vi "Dialog Condition Client.vi"() -> ()   [LabVIEW 2019, in "OPC UA Demo.lvlib"]
doc: "Demonstrates the use of the <B>OPC UA Dialog Condition</B> functionality as an OPC UA client."
uses:
  OPC UA Demo.lvlib
  <vilib>/OPCUA/controls/NodeIds.ctl
  <vilib>/OPCUA/controls/NodeId.ctl
  <vilib>/OPCUA/controls/Write Variant Request.ctl
  <vilib>/OPCUA/controls/Write Status.ctl
  <vilib>/OPCUA/client/Multiple Write Variant.vi
  <vilib>/OPCUA/NI OPC UA Client.lvlib
panel:
  in  "enable/disable":bool
  in  "source node ID":string="Notifier.Source Node"
  out "active":bool
  in  "condition node ID":string="ns=2;s=Notifier.Dialog Condition Node"
  in  "stop":bool
  in  "server endpoint URL":string="opc.tcp://localhost:49580"
  # "Overview: Demonstrates the use of the OPC UA Dialog Condition functionality as an OPC UA client.\nRequirements: \n1. LabVIEW OPC UA Toolkit\n2. Run this VI on RT targets or Windows\nInstructions:\n1. Specify the server endpoint URL generated by the server.\n2. Run the VI.\n3. Click enable/disable to enable/disable the dialog condition node."
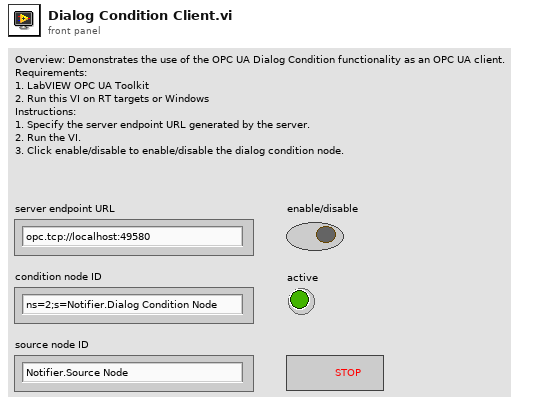
[diagram p1: front panel]
types:
  T1 = typedef "NodeIds.ctl" = T2[]
  T2 = typedef "NodeId.ctl" = string
  T3 = cluster{"message mode":enum16{"None", "Sign", "Sign and Encrypt"}, "security":enum16{"Basic256", "Basic128Rsa15"}}
  T4 = typedef "OPC UA Client Refnum.ctl" = refnum<k21>
  T5 = typedef "Subscription ID.ctl" = u32
  T6 = typedef "Write Variant Request.ctl" = cluster{"node ID":T2, "value":variant, "timestamp (current time)":timestamp, "node status":T7}
  T7 = typedef "Write Status.ctl" = u32
  T8 = typedef "Event Fields.ctl" = cluster{"condition node ID":T2, "condition type":T9, "source node ID/input node ID":T2, "event ID":string, "active":bool, "time":timestamp, "severity":u16, "quality":T10, "comment":string, "limit state":cluster{"high high state":bool, "high state":bool, "low state":bool, "low low state":bool}, "acked state":bool, "confirmed state":bool, "prompt":string}
  T9 = typedef "Condition Type.ctl" = enum16{"Dialog Condition", "Off-Normal Alarm", "Exclusive Level Alarm", "Exclusive Deviation Alarm", "Exclusive Rate of Change Alarm", "Nonexclusive Level Alarm", "Nonexclusive Deviation Alarm", "Nonexclusive Rate of Change Alarm", "Refresh Start Event", "Refresh End Event"}
  T10 = typedef "OPC UA StatusCode.ctl" = u32
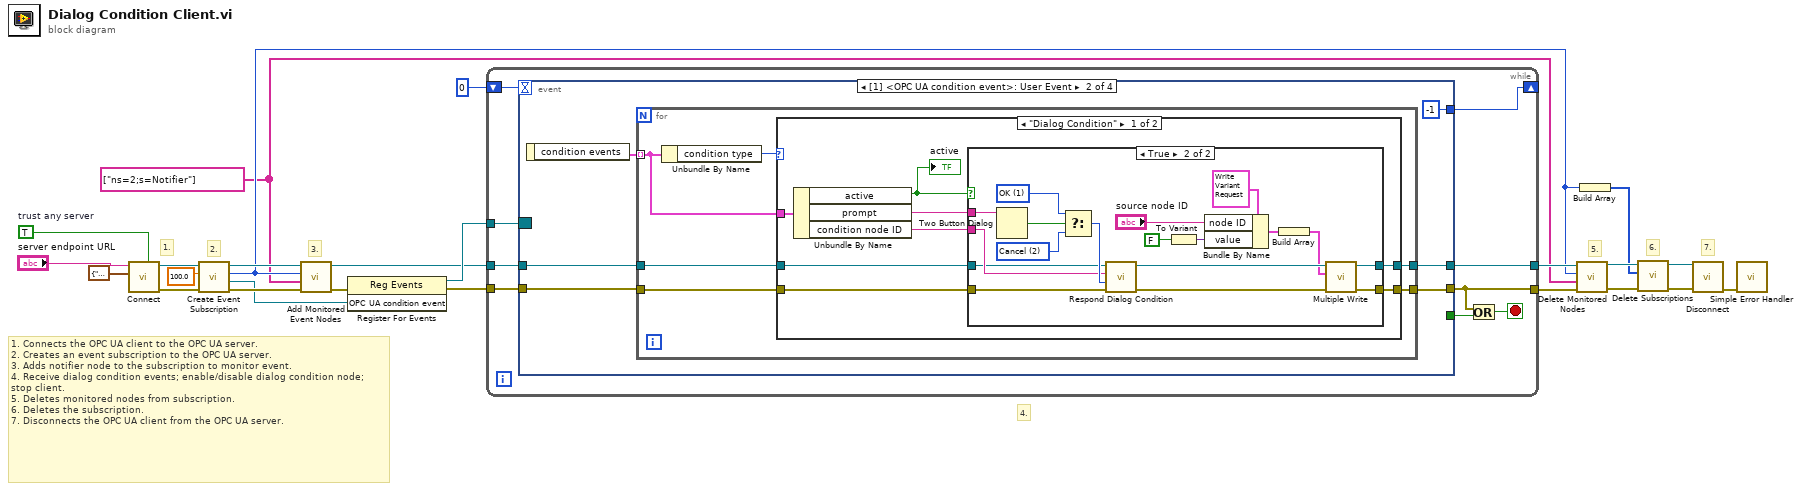
[diagram p0: block diagram]
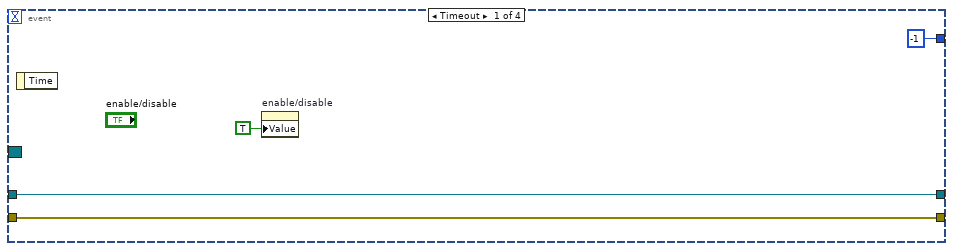
[diagram p2: hidden frame]
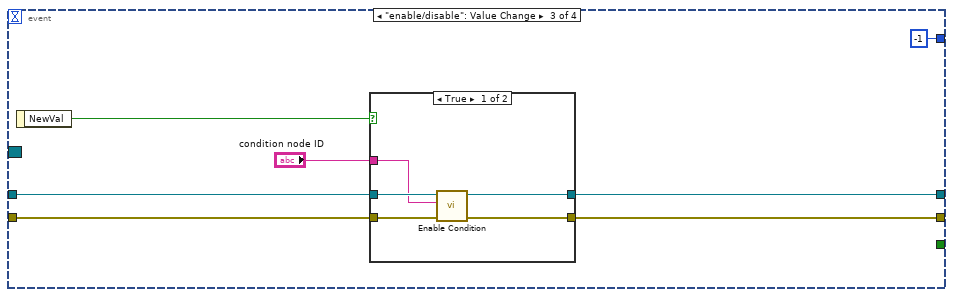
[diagram p5: hidden frame]
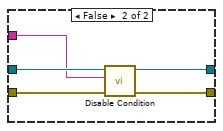
[diagram p6: hidden frame]
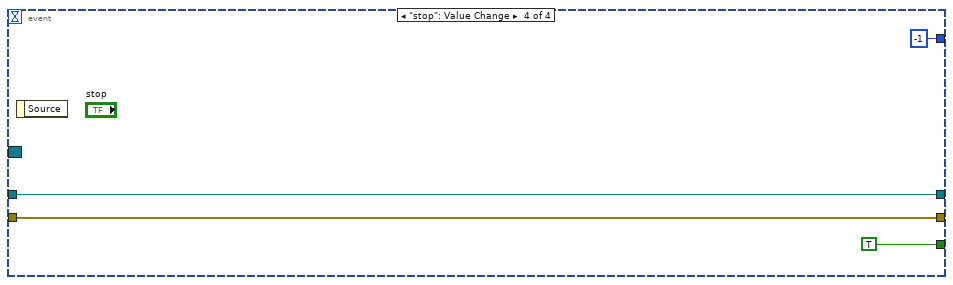
[diagram p7: hidden frame]
diagram:
  w1 = TRUE  # trust any server
  w3 = T1 ["ns=2;s=Notifier"] ("node IDs")
  # "6."
  # "5."
  # "7."
  # "4."
  # "3."
  # "2."
  # "1."
  # "1. Connects the OPC UA client to the OPC UA server. \n2. Creates an event subscription to the OPC UA server.\n3. Adds notifier node to the subscription to monitor event.\n4. Receive dialog condition events; enable/disable dialog condition node; stop client.\n5. Deletes monitored nodes from subscription.\n6. Deletes the subscription.\n7. Disconnects the OPC UA client from the OPC UA server."
  n1 = call <vilib>:"Connect.vi"("trust any server (F)"=w1, "security policy"=T3 {"message mode"=enum."None", "security"=enum."Basic256"}, "server endpoint URL"="server endpoint URL") -> ("error out"=w20:errorcluster, "OPC UA client refnum out"=w19:T4)  [unwired: 6 in, 1 out]
  n2 = call <vilib>:"Create Event Subscription.vi"("error in (no error)"=w20, "publishing interval (1000 ms)"=100.0 ("update rate (1000 ms)"), "OPC UA client refnum in"=w19) -> ("error out"=w24:errorcluster, "OPC UA condition event"=w18:refnum<user-event>, "subscription ID out"=w5:T5, "OPC UA client refnum out"=w7:T4)  [unwired: 4 in, 1 out]
  n3 = call <vilib>:"Add Monitored Event Nodes.vi"("error in (no error)"=w24, "node IDs"=w3, "subscription ID in"=w5, "OPC UA client refnum in"=w7) -> ("error out"=w23:errorcluster, "OPC UA client refnum out"=w4:T4)  [unwired: 4 in, 2 out]
  n4 = register-events(error in=w23, w18) -> (reference out=w16:refnum<event-registration>, error out=w14:errorcluster)  [unwired: 1 in]
  n5 = while {
    tunnel: w16 -> [w33]
    tunnel: w14 -> [w32]
    tunnel: [w29] -> w12
    tunnel: w4 -> [w31]
    tunnel: [w30] -> w13
    shift-right: [w26] -> _
    shift-left: 0 -> [w27]
    stop <- w28 stop-if-true
    n6 = event shown="[1] <OPC UA condition event>: User Event" {
      selector: w33 -> [_ _ _ _]
      dyn-events: _ -> [_ _ _ _]
      timeout: w27 -> [_ _ _ _]
      tunnel: w32 -> [w34 w40 w81 w99]
      tunnel: [w34 w43 w80 w99] -> w29
      tunnel: w31 -> [w37 w41 w86 w100]
      tunnel: [w37 w42 w85 w100] -> w30
      tunnel: [_ _ _ TRUE ("NewVal")] -> w25
      tunnel: [-1 -1 -1 -1] -> w26
      event Timeout {
        n7 = event-data() -> ()  [unwired: 1 in, 1 out]
        n8 = property on="enable/disable" class="Bool (strict)"("Value"=TRUE ("enable/disable")) -> ()  [unwired: 2 in, 2 out]
      }
      event User Event {
        n9 = event-data() -> ("condition events"=w39:T8[])  [unwired: 1 in]
        n10 = for {
          tunnel: [w49] -> w42
          tunnel: [w48] -> w43
          tunnel: w41 -> [w47]
          tunnel: w40 -> [w46]
          tunnel: w39 -> [w45] mode=indexing
          n11 = Unbundle By Name(w45) -> ("condition type"=w44:T9)
          n12 = case shown="\"Dialog Condition\"" w44 {
            tunnel: [w54 w79] -> w49
            tunnel: [w53 w78] -> w48
            tunnel: w47 -> [w52 w79]
            tunnel: w46 -> [w51 w78]
            tunnel: w45 -> [w50 _]
            frame "Dialog Condition" {
              n13 = Unbundle By Name(w50) -> ("active"=w57:bool, "prompt"=w56:string, "condition node ID"=w55:T2)
              "active" <- w57
              n14 = case shown="True" w57 {
                tunnel: [w59 w70] -> w54
                tunnel: [w58 w69] -> w53
                tunnel: w55 -> [_ w68]
                tunnel: w56 -> [_ w73]
                tunnel: w52 -> [w59 w61]
                tunnel: w51 -> [w58 w60]
                frame False {
                }
                frame True {
                  w75 = u16 2 items=["OK"=1, "Cancel"=2] ("response")
                  w76 = u16 1 items=["OK"=1, "Cancel"=2] ("response")
                  n15 = Two Button Dialog(message=w73) -> (T button?=w77:bool)  [unwired: 2 in]
                  n16 = Select(t=w76, s=w77, f=w75) -> (s? t:f=w74:u16)
                  n17 = call <vilib>:"Respond Dialog Condition.vi"("error in (no error)"=w60, "response"=w74, "condition node ID"=w68, "OPC UA client refnum in"=w61) -> ("error out"=w71:errorcluster, "OPC UA client refnum out"=w72:T4)  [unwired: 5 in, 1 out]
                  n18 = To Variant(anything=FALSE ("value")) -> (Variant=w63:variant)
                  n19 = Bundle By Name(cluster=T6 {"node ID"="", "value"=variant, "timestamp (current time)"=timestamp(0 s since 1904-01-01), "node status"=0} ("request"), "node ID"="source node ID", "value"=w63) -> (w66:T6)
                  n20 = Build Array(w66) -> (w65:T6[])
                  n21 = call-poly <vilib>:"Multiple Write.vi"("error in (no error)"=w71, "requests"=w65, "OPC UA client refnum in"=w72) -> ("error out"=w69:errorcluster, "OPC UA client refnum out"=w70:T4)  [unwired: 5 in, 2 out]
                }
              }
            }
            frame "Refresh Start Event", Default {
            }
          }
        }
      }
      event "enable/disable": Value Change {
        n22 = event-data() -> ("NewVal"=w82:bool)  [unwired: 1 in]
        n23 = case shown="True" w82 {
          tunnel: w86 -> [w91 w96]
          tunnel: "condition node ID" -> [w90 w95]
          tunnel: [w89 w94] -> w85
          tunnel: [w88 w93] -> w80
          tunnel: w81 -> [w87 w92]
          frame True {
            n24 = call <vilib>:"Enable Condition.vi"("error in (no error)"=w87, "condition node ID"=w90, "OPC UA client refnum in"=w91) -> ("error out"=w88:errorcluster, "OPC UA client refnum out"=w89:T4)  [unwired: 6 in, 1 out]
          }
          frame False {
            n25 = call <vilib>:"Disable Condition.vi"("error in (no error)"=w92, "condition node ID"=w95, "OPC UA client refnum in"=w96) -> ("error out"=w93:errorcluster, "OPC UA client refnum out"=w94:T4)  [unwired: 6 in, 1 out]
          }
        }
      }
      event "stop": Value Change {
        n26 = event-data() -> ()  [unwired: 1 in, 1 out]
      }
    }
    n27 = Or(x=w29, y=w25) -> (x .or. y?=w28:bool)
  }
  n28 = call <vilib>:"Delete Monitored Nodes.vi"("error in (no error)"=w12, "node IDs"=w3, "subscription ID in"=w5, "OPC UA client refnum in"=w13) -> ("error out"=w9:errorcluster, "OPC UA client refnum out"=w11:T4)  [unwired: 3 in, 3 out]
  n29 = Build Array(w5) -> (w6:T5[])
  n30 = call <vilib>:"Delete Subscriptions.vi"("error in (no error)"=w9, "subscription IDs"=w6, "OPC UA client refnum in"=w11) -> ("error out"=w8:errorcluster, "OPC UA client refnum out"=w10:T4)  [unwired: 6 in, 1 out]
  n31 = call <vilib>:"Disconnect.vi"("error in (no error)"=w8, "OPC UA client refnum in"=w10) -> ("error out"=w15:errorcluster)  [unwired: 9 in]
  n32 = call <vilib>:"Simple Error Handler.vi"("error in (no error)"=w15) -> ()  [unwired: 4 in, 5 out]
